vi "Connect.vi"(8 "error in (no error)":errorcluster, 10 "Connection list in":string, 11 "Test Switch Consumer in":refnum<class "Test Switch Consumer.lvclass">) -> (0 "error out":errorcluster, 3 "Test Switch Consumer out":refnum<class "Test Switch Consumer.lvclass">)   [LabVIEW 2027, in "Test Switch Consumer.lvclass"]
uses:
  Test Switch Consumer.lvclass
  Message String Action.ctl
  Message List Action.ctl
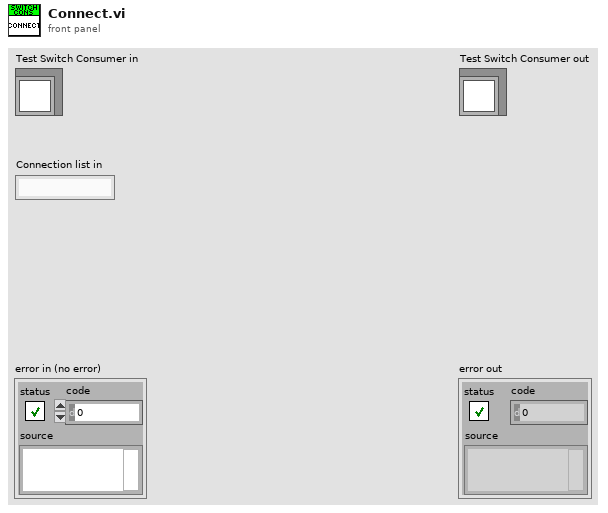
[diagram p1: front panel]
types:
  T1 = typedef "Message List Action.ctl" = enum16{"Get", "Add", "Reset"}
  T2 = typedef "Message String Action.ctl" = enum16{"Get String", "Set String", "Reset"}
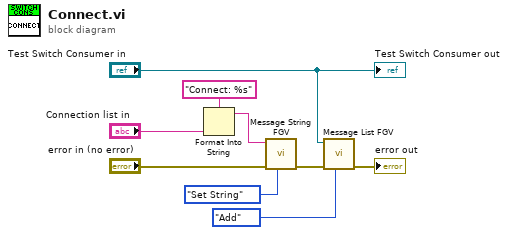
[diagram p0: block diagram]
diagram:
  n1 = Format Into String(format string="Connect: %s", "Connection list in") -> (resulting string=w6:string)  [unwired: 2 in, 1 out]
  n2 = call "Message String FGV.vi"("Action"=Message_String_Action."Set String", "error in (no error)"="error in (no error)", "Message String"=w6) -> ("error out"=w4:errorcluster)  [unwired: 7 in, 1 out]
  n3 = call "Message List FGV.vi"("Action (Get)"=Message_List_Action."Add", "error in (no error)"=w4, "Message Object"="Test Switch Consumer in") -> ("error out"=→"error out":errorcluster)  [unwired: 7 in, 1 out]
  "Test Switch Consumer out" <- "Test Switch Consumer in"
